vi "Intake_Globals.vi"() -> ()   [LabVIEW 2019]
uses:
  Intake_Cluster.ctl
  Intake_States.ctl
  Utility_VIs/Basic_Motor_Modes.ctl
  <vilib>/Rock Robotics/WPI/Solenoid/WPI_SolenoidValue.ctl
panel:
  in  "Pneumatic_State":T1=enum."Forward"
  in  "Motor_Mode":T2
  in  "Motor Output":dbl
  out "Intake_Running":bool
  in  "Intake_Left":string="Intake_Left"
  in  "Intake_Right":string="Intake_Right"
  in  "Intake_Execute_Notifier":refnum<notifier>
  in  "Intake_Set_Notifier":refnum<notifier>
  in  "Intake_Execute_Ref":string="Intake_Execute_Ref"
  in  "Intake_Set_Ref":string="Intake_Set_Ref"
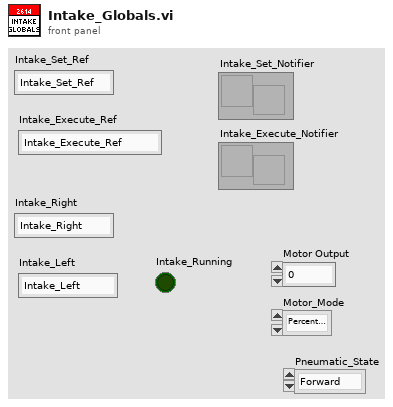
[diagram p1: front panel]
types:
  T1 = typedef "WPI_SolenoidValue.ctl" = enum16{"Off", "On", "Forward", "Reverse"}
  T2 = typedef "Basic_Motor_Modes.ctl" = enum16{"Percent_Voltage", "Speed_Control", "Position_Control", "Current"}
diagram:
